vi "subscription test.vi"() -> ()   [LabVIEW 2013, in "tdms logger tests.lvlib"]
uses:
  tdms logger tests.lvlib
  configuration/TDMS datalogger configuration.lvclass
  <vilib>/NI/Tag Bus Module Framework/channel/TBM channel.lvclass
panel:
  out "error out":errorcluster
  out "local OK":bool
  out "remote OK":bool
  out "ALL channels OK":bool
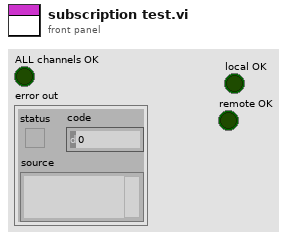
[diagram p1: front panel]
types:
  T1 = typedef "TBM module configuration.lvclass/channel reservation.ctl" = cluster{"local channel":refnum<class "TBM channel.lvclass">, "remote channel":refnum<class "TBM channel.lvclass">}
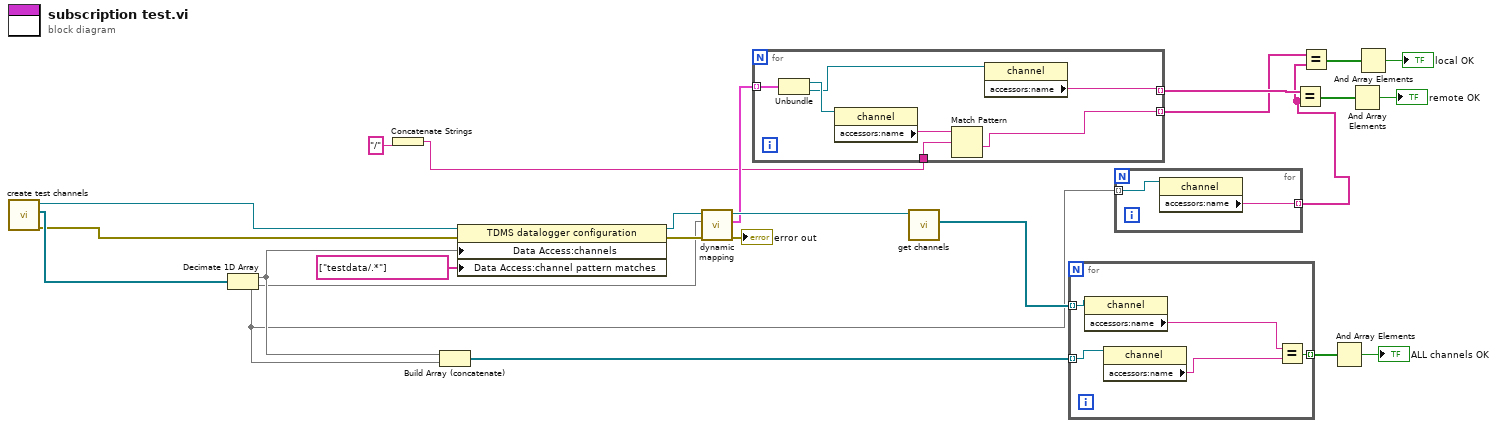
[diagram p0: block diagram]
diagram:
  n1 = call "create test channels.vi"() -> ("error out"=w1:errorcluster, "chans"=w2:refnum<class "TBM channel.lvclass">[], "TDMS datalogger configuration out"=w3:refnum<class "TDMS datalogger configuration.lvclass">)  [unwired: 8 in, 1 out]
  n2 = Decimate 1D Array(w2) -> (w18:refnum<class "TBM channel.lvclass">[], w4:refnum<class "TBM channel.lvclass">[])
  n3 = Concatenate Strings("/" ("string")) -> (w7:string)
  n4 = Build Array (concatenate)(w18, w4) -> (w17:refnum<class "TBM channel.lvclass">[])
  n5 = property class="TDMS datalogger configuration"(reference=w3, error in=w1, "Data Access:channels"=w18, "Data Access:channel pattern matches"=string[] ["testdata/.*"] ("channel pattern matches")) -> (reference out=w22:refnum<class "TDMS datalogger configuration.lvclass">, error out=w23:errorcluster)
  n6 = call-dynamic "dynamic mapping.vi"("error in"=w23, "channels available"=w4, "module configuration in"=w22) -> ("error out"=→"error out":errorcluster, "reservations"=w14:T1[], "module configuration out"=w20:refnum<class "TDMS datalogger configuration.lvclass">)  [unwired: 6 in]
  n7 = for {
    tunnel: w14 -> [w31] mode=indexing
    tunnel: [w26] -> w11 mode=indexing
    tunnel: [w27] -> w8 mode=indexing
    tunnel: w7 -> [w29]
    n8 = Unbundle(w31) -> ("local channel"=w30:refnum<class "TBM channel.lvclass">, "remote channel"=w25:refnum<class "TBM channel.lvclass">)
    n9 = property class="channel"(reference=w30) -> ("accessors:name"=w28:string)  [unwired: 1 in, 2 out]
    n10 = Match Pattern(string=w28, regular expression=w29) -> (after substring=w27:string)  [unwired: 1 in, 3 out]
    n11 = property class="channel"(reference=w25) -> ("accessors:name"=w26:string)  [unwired: 1 in, 2 out]
  }
  n12 = call-dynamic "get channels.vi"("module configuration in"=w20) -> ("channels"=w19:refnum<class "TBM channel.lvclass">[])  [unwired: 9 in, 1 out]
  n13 = for {
    tunnel: w19 -> [w35] mode=indexing
    tunnel: w17 -> [w34] mode=indexing
    tunnel: [w36] -> w16 mode=indexing
    n14 = property class="channel"(reference=w35) -> ("accessors:name"=w32:string)  [unwired: 1 in, 2 out]
    n15 = property class="channel"(reference=w34) -> ("accessors:name"=w33:string)  [unwired: 1 in, 2 out]
    n16 = Equal?(x=w32, y=w33) -> (x = y?=w36:bool)
  }
  n17 = for {
    tunnel: [w38] -> w5 mode=indexing
    tunnel: w4 -> [w37] mode=indexing
    n18 = property class="channel"(reference=w37) -> ("accessors:name"=w38:string)  [unwired: 1 in, 2 out]
  }
  n19 = Equal?(x=w11, y=w5) -> (x = y?=w12:bool[])
  n20 = Equal?(x=w8, y=w5) -> (x = y?=w10:bool[])
  n21 = And Array Elements(Boolean array=w16) -> (logical AND=→"ALL channels OK":bool)
  n22 = And Array Elements(Boolean array=w12) -> (logical AND=→"remote OK":bool)
  n23 = And Array Elements(Boolean array=w10) -> (logical AND=→"local OK":bool)
